vi "Channel_discard.vi"(4 "DIscard Channel Info":i32[](array[numeric]), 11 "Array":dbl[][](array[numeric])) -> (3 "array w/ subset deleted":dbl[][](array[numeric]))   [LabVIEW 2014]
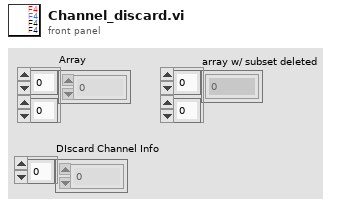
[diagram p1: front panel]
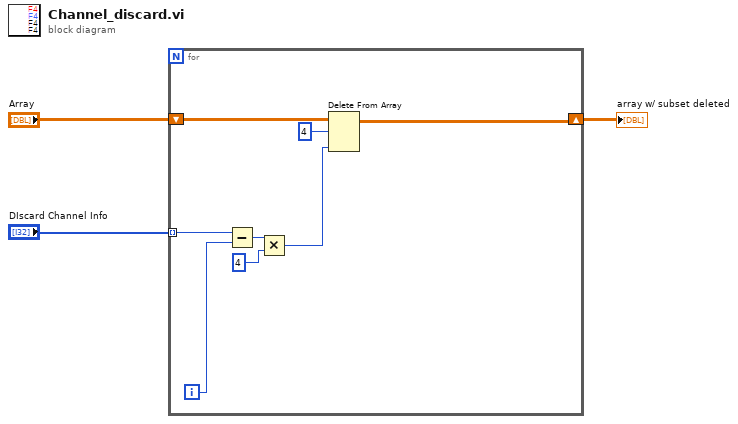
[diagram p0: block diagram]
diagram:
  n1 = for {
    tunnel: "DIscard Channel Info" -> [w8] mode=indexing
    shift-right: [w9] -> w1
    shift-left: "Array" -> [w10]
    i -> [w7]
    n2 = Subtract(x=w8, y=w7) -> (x-y=w6:i32)
    n3 = Multiply(x=w6, y=4 ("disabled index (col)")) -> (x*y=w4:i32)
    n4 = Delete From Array(array=w10, length=4, index (col)=w4) -> (array with subset deleted=w9:dbl[][])  [unwired: 1 in, 1 out]
  }
  "array w/ subset deleted" <- w1
